vi "Read DI Group.vi"(8 "error in (no error)":errorcluster, 10 "Write/Read 1 DI Index":T2[](array[typedef]), 11 "dCVT DAQDict":T1) -> (0 "error out":errorcluster, 2 "DIO out":bool[](array[boolean]), 3 "dCVT DAQDict out":T1)   [LabVIEW 2020, in "DAQDict.lvlib"]
uses:
  DAQDict.lvlib
  support/IONameNode--cluster.ctl
  support/BRS_DI - New.ctl
  <vilib>/TELLC/Dynamic CVT API/TD Dynamic CVT DVR--ref.ctl
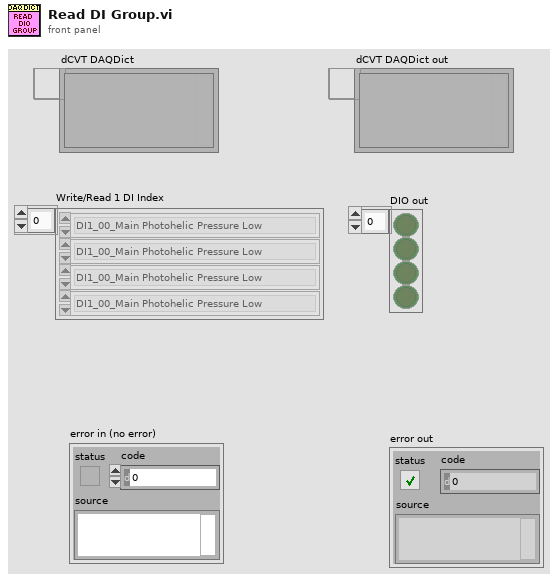
[diagram p1: front panel]
types:
  T1 = typedef "TD Dynamic CVT DVR--ref.ctl" = refnum<data-value>
  T2 = typedef "BRS_DI - New.ctl" = enum16{"DI1_00_Main Photohelic Pressure Low", "DI1_01_Main Photohelic Pressure High", "DI1_02_Main E-Stop Circuit OK", "DI1_03_EMO Circuit OK", "DI1_04_Nitrogen Top Valve Open", "DI1_05_Nitrogen Bottom Valve Open", "DI1_06_Nitrogen Pressure OK", "DI1_07_CDA Pressure OK", "DI1_08_Vacuum OK", "DI1_09_Aligner Home", "DI1_10_Aligner Reticle Present", "DI1_11_Main Door Interlock Solenoid Closed", "DI1_12_Main Door Closed", "DI1_13_Main Robot $ALARM_STOP", "DI1_14_Main Robot $IN_HOME", "DI1_15_Main Robot $PERI_RDY", "DI1_16_Main Robot $TCP_OPEN", "DI1_17_Main End Eff Open", "DI1_18_Main End Eff Closed", "DI1_19_Main Reticle Presence sensor-Arm-Right", "DI1_20_Spare_1", "DI1_21_Main Reticle Presence sensor-Arm-Left", "DI1_22_EXP1 XFR Reticle Present", "DI1_23_EXP2 XFR Reticle Present", "DI1_24_Main Robot $EXT (External Mode ON)", "DI1_25_Main Robot $PRO_ACT (Program Active)", "DI1_26_Main Robot $PRO_MOVE (Motion Active)", "DI1_27_Main Robot Spare1", "DI1_28_Main Robot Spare2", "DI1_29_Main Robot Spare3", "DI1_30_Spare_2", "DI1_31_Spare_3", "DI2_00_ASML_RSP LP 1 Pod Presence", "DI2_01_Spare_4", "DI2_02_ASML_RSP LP 2 Pod Presence", "DI2_03_Spare_5", "DI2_04_ASML_RSP LP 3 Pod Presence", "DI2_05_Spare_6", "DI2_06_Spare_7", "DI2_07_Manual Loadport 1 Pod Present", "DI2_08_Manual Loadport 1 Pod Capture", "DI2_09_Manual Loadport 1 Arm in Open Position", "DI2_10_Manual Loadport 1 Arm in Closed Position", "DI2_11_Manual Loadport 1 Lid Capture", "DI2_12_Manual Loadport 1 Door Closed", "DI2_13_Manual Loadport 1 Reticle Present", "DI2_14_Manual Loadport 1 Lid Present on Arm", "DI2_15_MLP Spare Input", "DI2_16_Pod Buffer Inbound Pod Present", "DI2_17_Pod Buffer Outbound Pod Present", "DI2_18_Pod Buffer Door Closed", "DI2_19_Pod Buffer Light Curtain OK", "DI2_20_Pod Buffer Light Curtain Misc Input", "DI2_21_Pod Buffer Gripper Pod Present", "DI2_22_Pod Buffer Gripper open", "DI2_23_Pod Buffer Gripper closed", "DI2_24_FFU Pressure sensor 1", "DI2_25_FFU Pressure sensor 2", "DI2_26_FFU Pressure sensor 3", "DI2_27_FFU Pressure sensor 4", "DI2_28_FFU Pressure sensor 5", "DI2_29_FFU Pressure sensor 6", "DI2_30_FFU Pressure sensor 7", "DI2_31_FFU Pressure sensor 8", "DI3_00_Exp1 Photohelic Pressure Low", "DI3_01_Exp1 Photohelic Pressure High", "DI3_02_Main E-Stop Circuit OK", "DI3_03_Spare_1", "DI3_04_Exp1 Door Interlock Solenoid Closed", "DI3_05_Exp1 Door Closed", "DI3_06_Spare_2", "DI3_07_Spare_3", "DI3_08_Spare_4", "DI3_09_Spare_5", "DI3_10_Exp1 End Eff Open", "DI3_11_Exp1 End Eff Closed", "DI3_12_Exp1 Reticle Presence sensor-Arm-Right", "DI3_13_Exp1 Robot $ALARM_STOP", "DI3_14_Exp1 Robot $IN_HOME", "DI3_15_Exp1 Robot $PERI_RDY", "DI3_16_Exp1 Robot $TCP_OPEN", "DI3_17_Exp1 Reticle Presence sensor-Arm-Left", "DI3_18_Exp1 FFU Pressure sensor 1", "DI3_19_Exp1 FFU Pressure sensor 2", "DI3_20_Exp1 FFU Pressure sensor 3", "DI3_21_Exp1 FFU Pressure sensor 4", "DI3_22_Exp1 FFU Pressure sensor 5", "DI3_23_Exp1 FFU Pressure sensor 6", "DI3_24_Exp1 Robot $EXT (External Mode ON)", "DI3_25_Exp1 Robot $PRO_ACT (Program Active)", "DI3_26_Exp1 Robot $PRO_MOVE (Motion Active)", "DI3_27_Exp1 FFU Pressure sensor 7", "DI3_28_Exp1 FFU Pressure sensor 8", "DI3_29_Exp1 output Spare 1", "DI3_30_Exp1 output Spare 2", "DI3_31_Exp1 output Spare 3"}
  T3 = typedef "IONameNode--cluster.ctl" = cluster{"IOName":string, "value":bool, "IO Type":enum16{"N/A", "DI", "DO"}, "TaskID":string, "data Idx":i32}
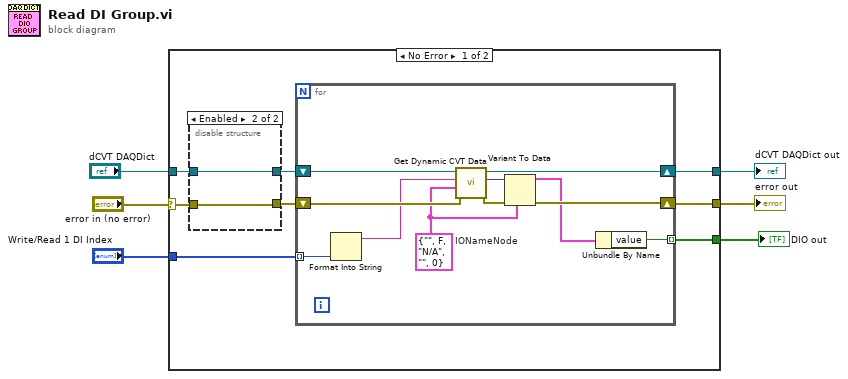
[diagram p0: block diagram]
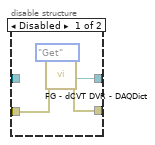
[diagram p2: hidden frame]
diagram:
  n1 = case shown="No Error" "error in (no error)" {
    selector: "error in (no error)" -> [w13 w33]
    tunnel: [w11 w33] -> w6
    tunnel: "Write/Read 1 DI Index" -> [w12 _]
    tunnel: [w10 _] -> w3
    tunnel: [w9 w32] -> w2
    tunnel: "dCVT DAQDict" -> [w7 w32]
    frame No Error {
      n2 = disable-structure shown="Enabled" {
        disable-tunnel: [w17 w19] -> w14
        disable-tunnel: w13 -> [w16 w19]
        disable-tunnel: [w15 w20] -> w8
        disable-tunnel: w7 -> [_ w20]
        frame Disabled {
          n3 = call "FG - dCVT DVR - DAQDict.vi"("error in (no error)"=w16, "Action (Get)"=enum16{"Init", "Get", "Set"}."Get") -> ("dCVT DAQDict out"=w15:T1, "error out"=w17:errorcluster)  [unwired: 7 in]
        }
        frame Enabled {
        }
      }
      n4 = for {
        shift-right: [w28] -> w9
        shift-left: w8 -> [w31]
        shift-right: [w27] -> w11
        shift-left: w14 -> [w30]
        tunnel: w12 -> [w29] mode=indexing
        tunnel: [w21] -> w10 mode=indexing
        w24 = T3 {"IOName"="", "value"=FALSE, "IO Type"=enum."N/A", "TaskID"="", "data Idx"=0}  # IONameNode
        n5 = Format Into String(w29) -> (resulting string=w23:string)  [unwired: 3 in, 1 out]
        n6 = call <vilib>:"Get Dynamic CVT Data.vi"("error in (no error)"=w30, "default value (empty variant)"=w24, "DataName"=w23, "dCVT DVR"=w31) -> ("error out"=w25:errorcluster, "value"=w26:variant, "dCVT DVR out"=w28:T1)  [unwired: 4 in, 1 out]
        n7 = Variant To Data(error in=w25, type=w24, Variant=w26) -> (data=w22:T3, error out=w27:errorcluster)
        n8 = Unbundle By Name(w22) -> ("value"=w21:bool)
      }
    }
    frame Error {
    }
  }
  "DIO out" <- w3
  "error out" <- w6
  "dCVT DAQDict out" <- w2
